vi "Is Filled.vi"(8 "error in (no error)":errorcluster, 11 "Tool Rectangle in":refnum<class "Tool Rectangle.lvclass">) -> (0 "error out":errorcluster, 2 "x != y?":bool, 3 "Tool Rectangle out":refnum<class "Tool Rectangle.lvclass">)   [LabVIEW 2019, in "Tool Rectangle.lvclass"]
uses:
  Tool Rectangle.lvclass
  Parse/Rectangle/Rectangle.lvclass/Rectangle.ctl
  Parse/CSSProperties/CSSProperties.lvclass/CSSProperties.ctl
  Parse/CSSProperties/CSSProperties.lvclass
  Parse/Rectangle/Rectangle.lvclass
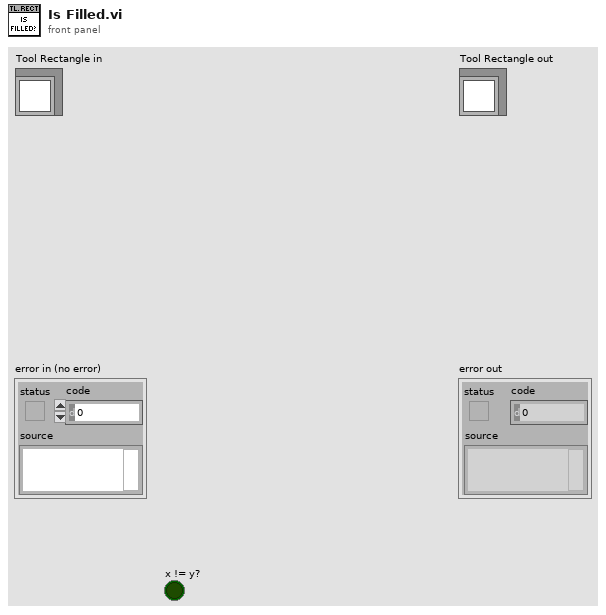
[diagram p1: front panel]
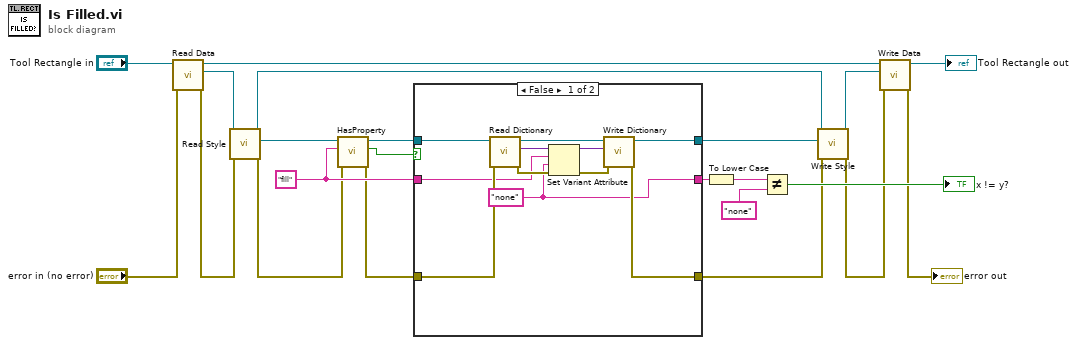
[diagram p0: block diagram]
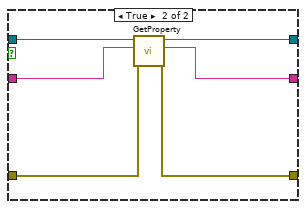
[diagram p2: hidden frame]
diagram:
  w21 = "fill" ("Property")
  n1 = call-dynamic "Read Data.vi"("error in (no error)"="error in (no error)", "Tool Rectangle in"="Tool Rectangle in") -> ("error out"=w8:errorcluster, "Rectangle.lvclass"=w13:refnum<class "Rectangle.lvclass">, "Tool Rectangle out"=w7:refnum<class "Tool Rectangle.lvclass">)  [unwired: 7 in]
  n2 = call "Read Style.vi"("error in (no error)"=w8, "Rectangle in"=w13) -> ("error out"=w1:errorcluster, "CSSProperties.lvclass"=w12:refnum<class "CSSProperties.lvclass">, "Rectangle out"=w5:refnum<class "Rectangle.lvclass">)  [unwired: 7 in]
  n3 = call "HasProperty.vi"("error in (no error)"=w1, "Property"=w21, "CSSProperties in"=w12) -> ("error out"=w16:errorcluster, "Exists?"=w22:bool, "CSSProperties out"=w20:refnum<class "CSSProperties.lvclass">)  [unwired: 6 in]
  n4 = case shown="False" w22 {
    tunnel: [w30 w39] -> w11
    tunnel: [w23 w35] -> w19
    tunnel: w20 -> [w29 w38]
    tunnel: w21 -> [w24 w34]
    tunnel: [w28 w37] -> w10
    tunnel: w16 -> [w27 w36]
    frame False {
      w23 = "none" ("Value")
      n5 = call "Read Dictionary.vi"("error in (no error)"=w27, "CSSProperties in"=w29) -> ("error out"=w25:errorcluster, "Dictionary"=w32:variant, "CSSProperties out"=w31:refnum<class "CSSProperties.lvclass">)  [unwired: 7 in]
      n6 = Set Variant Attribute(Variant=w32, name=w24, value=w23, error in=w25) -> (Variant out=w33:variant, error out=w26:errorcluster)  [unwired: 1 out]
      n7 = call "Write Dictionary.vi"("error in (no error)"=w26, "Dictionary"=w33, "CSSProperties in"=w31) -> ("error out"=w28:errorcluster, "CSSProperties out"=w30:refnum<class "CSSProperties.lvclass">)  [unwired: 7 in]
    }
    frame True {
      n8 = call "GetProperty.vi"("error in (no error)"=w36, "Property"=w34, "CSSProperties in"=w38) -> ("error out"=w37:errorcluster, "Value"=w35:string, "CSSProperties out"=w39:refnum<class "CSSProperties.lvclass">)  [unwired: 6 in]
    }
  }
  n9 = To Lower Case(string=w19) -> (all lower case string=w18:string)
  n10 = Not Equal?(x=w18, y="none") -> (x != y?=→"x != y?":bool)
  n11 = call "Write Style.vi"("error in (no error)"=w10, "CSSProperties.lvclass"=w11, "Rectangle in"=w5) -> ("error out"=w3:errorcluster, "Rectangle out"=w4:refnum<class "Rectangle.lvclass">)  [unwired: 7 in]
  n12 = call-dynamic "Write Data.vi"("error in (no error)"=w3, "Rectangle.lvclass"=w4, "Tool Rectangle in"=w7) -> ("error out"=→"error out":errorcluster, "Tool Rectangle out"=→"Tool Rectangle out":refnum<class "Tool Rectangle.lvclass">)  [unwired: 7 in]
